vi "Evaluate Part 1.vi"() -> ()   [LabVIEW 2020]
uses:
  Proto/Group.lvclass
panel:
  out "sum":u64
  in  "Input":string
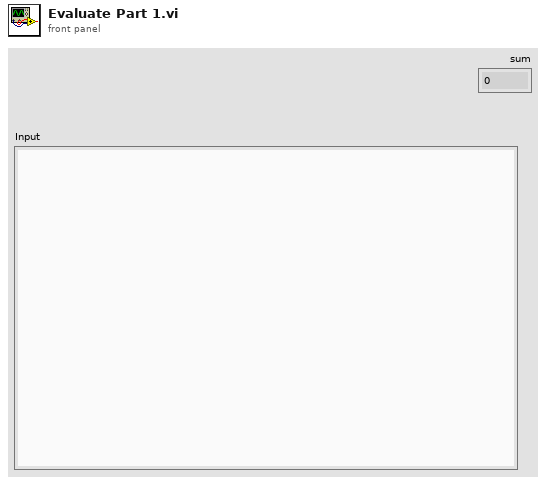
[diagram p1: front panel]
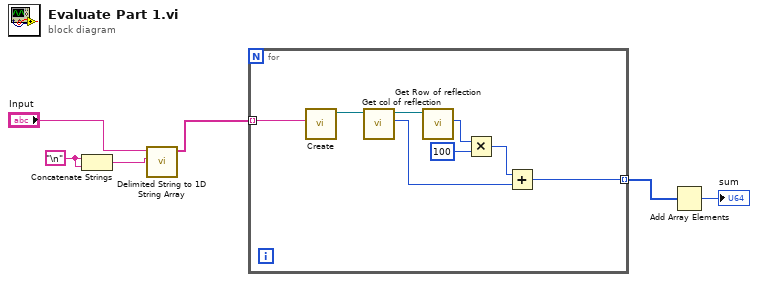
[diagram p0: block diagram]
diagram:
  w2 = "\n"
  n1 = Concatenate Strings(w2, w2) -> (w3:string)
  n2 = call <vilib>:"Delimited String to 1D String Array.vi"("delimiter"=w3, "delimited string"="Input") -> ("string array"=w5:string[])  [unwired: 9 in]
  n3 = for {
    tunnel: w5 -> [w8] mode=indexing
    tunnel: [w7] -> w4 mode=indexing
    n4 = call "Create.vi"("Input"=w8) -> ("Proto"=w14:refnum<class "Group.lvclass">)  [unwired: 9 in, 1 out]
    n5 = call "Get col of reflection.vi"("Proto in"=w14) -> ("Numeric"=w9:u64, "Proto out"=w13:refnum<class "Group.lvclass">)  [unwired: 8 in, 1 out]
    n6 = call "Get Row of reflection.vi"("Proto in"=w13) -> ("Numeric"=w12:u64)  [unwired: 8 in, 2 out]
    n7 = Multiply(x=w12, y=u64 100) -> (x*y=w10:u64)
    n8 = Add(x=w10, y=w9) -> (x+y=w7:u64)
  }
  n9 = Add Array Elements(numeric array=w4) -> (sum=→"sum":u64)
